vi "Get Component by Product Name.vi"(0 "Build Analyzer in":refnum<class "Build Analyzer.lvclass">, 5 "Component's Product Name":string, 11 "error in (no error)":errorcluster) -> (4 "Build Analyzer out":refnum<class "Build Analyzer.lvclass">, 6 "Component":refnum<class "Component.lvclass">, 8 "Found":bool, 15 "error out":errorcluster)   [LabVIEW 2017, in "CL_G3_VIComponentBuilder.lvlib" / "Build Analyzer.lvclass"]
doc: "Returns a compoent by its pretty print product name."
uses:
  Build Analyzer.lvclass
  Components/Component.lvclass
  Build Analyzer.lvclass/Build Analyzer.ctl
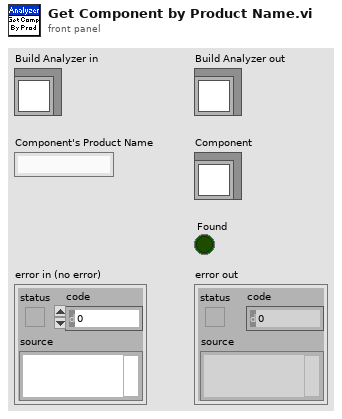
[diagram p1: front panel]
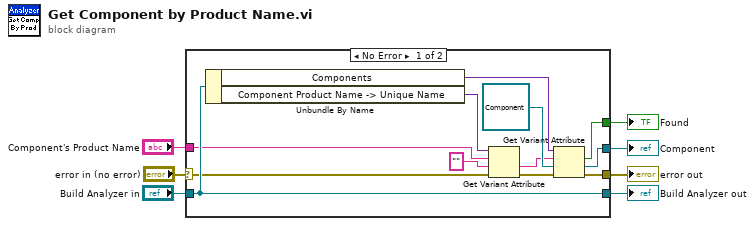
[diagram p0: block diagram]
diagram:
  n1 = case shown="No Error" "error in (no error)" {
    selector: "error in (no error)" -> [w10 w21]
    tunnel: [w8 w21] -> w6
    tunnel: [w19 w20] -> w4
    tunnel: "Build Analyzer in" -> [w19 w20]
    tunnel: "Component's Product Name" -> [w13 _]
    tunnel: [w16 _] -> w2
    tunnel: [w15 _] -> w1
    frame No Error {
      n2 = Unbundle By Name(w19) -> ("Components"=w18:variant, "Component Product Name -> Unique Name"=w14:variant)
      n3 = Get Variant Attribute(Variant=w14, name=w13, default value (empty Variant)="" ("Component's Product Name"), error in=w10) -> (value=w11:string, error out=w9:errorcluster)  [unwired: 2 out]
      n4 = Get Variant Attribute(Variant=w18, name=w11, default value (empty Variant)=refnum<class "Component.lvclass"> refnum ("Component"), error in=w9) -> (found=w15:bool, value=w16:refnum<class "Component.lvclass">, error out=w8:errorcluster)  [unwired: 1 out]
    }
    frame Error {
    }
  }
  "error out" <- w6
  "Build Analyzer out" <- w4
  "Component" <- w2
  "Found" <- w1
